vi "VAI Read Board Info.vi"(10 "pInfo":T1, 11 "DevIndex":i32) -> (2 "pInfo out":T1, 3 "function return":i32)   [LabVIEW 2010, in "ControlADC.lvlib"]
doc: "int WINAPI VAI_ReadBoardInfo(int DevIndex,PVAI_BOARD_INFO pInfo);"
uses:
  ControlADC.lvlib
  ControlADC/Ginkgo_Driver.dll
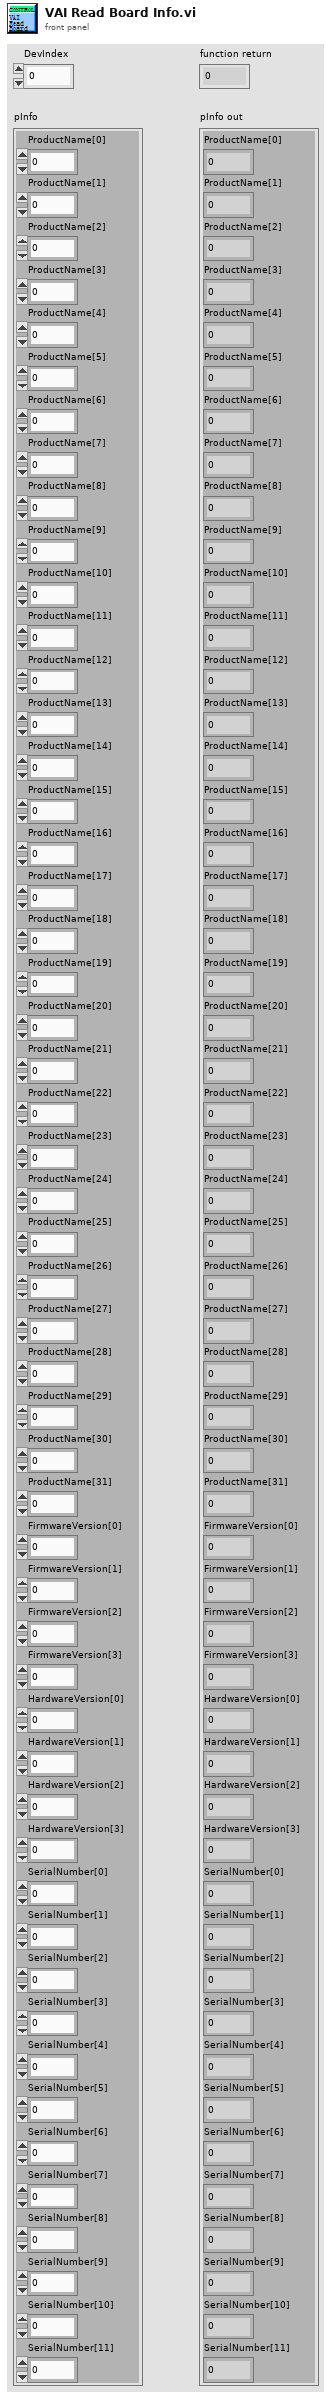
[diagram p1: front panel]
types:
  T1 = cluster{"ProductName[0]":u8, "ProductName[1]":u8, "ProductName[2]":u8, "ProductName[3]":u8, "ProductName[4]":u8, "ProductName[5]":u8, "ProductName[6]":u8, "ProductName[7]":u8, "ProductName[8]":u8, "ProductName[9]":u8, "ProductName[10]":u8, "ProductName[11]":u8, "ProductName[12]":u8, "ProductName[13]":u8, "ProductName[14]":u8, "ProductName[15]":u8, "ProductName[16]":u8, "ProductName[17]":u8, "ProductName[18]":u8, "ProductName[19]":u8, "ProductName[20]":u8, "ProductName[21]":u8, "ProductName[22]":u8, "ProductName[23]":u8, "ProductName[24]":u8, "ProductName[25]":u8, "ProductName[26]":u8, "ProductName[27]":u8, "ProductName[28]":u8, "ProductName[29]":u8, "ProductName[30]":u8, "ProductName[31]":u8, "FirmwareVersion[0]":u8, "FirmwareVersion[1]":u8, "FirmwareVersion[2]":u8, "FirmwareVersion[3]":u8, "HardwareVersion[0]":u8, "HardwareVersion[1]":u8, "HardwareVersion[2]":u8, "HardwareVersion[3]":u8, "SerialNumber[0]":u8, "SerialNumber[1]":u8, "SerialNumber[2]":u8, "SerialNumber[3]":u8, "SerialNumber[4]":u8, "SerialNumber[5]":u8, "SerialNumber[6]":u8, "SerialNumber[7]":u8, "SerialNumber[8]":u8, "SerialNumber[9]":u8, "SerialNumber[10]":u8, "SerialNumber[11]":u8}
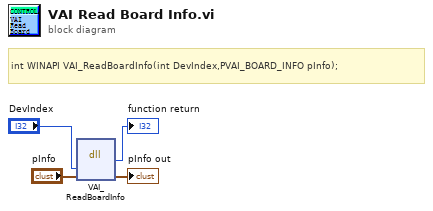
[diagram p0: block diagram]
diagram:
  # "int WINAPI VAI_ReadBoardInfo(int DevIndex,PVAI_BOARD_INFO pInfo);"
  n1 = dll-call lib="E:/Project/vt_ginkgo/truck/Ginkgo Driver/vs2010/Ginkgo_USB-I2C&SPI&CAN_API_v2.0.3.3/lib/labview_32bit/ControlADC/Ginkgo_Driver.*" fn="VAI_ReadBoardInfo"("DevIndex"="DevIndex", "pInfo"="pInfo") -> (→"function return":i32, "pInfo"=→"pInfo out":T1)  [unwired: 4 in, 2 out]
